vi "Receive Panel Close Event.vi"(8 "error in (no error)":errorcluster, 10 "PanelCloseMsg":refnum<class "PanelCloseMsg.lvclass">, 11 "OneButtonDialogBox in":refnum<class "OneButtonDialogBox.lvclass">) -> (0 "error out":errorcluster, 3 "OneButtonDialogBox out":refnum<class "OneButtonDialogBox.lvclass">)   [LabVIEW 2015, in "OneButtonDialogBox.lvlib" / "OneButtonDialogBox.lvclass"]
doc: "<License>\nCopyright © 2017 Composed Systems, LLC | All rights reserved\nwww.composed.io\n\nAuthor: Ethan Stern <ethan.stern@composed.io>\n\nThis software is provided \"AS IS\" WITHOUT WARRANTIES, either express or implied, AND IS FOR EDUCATIONAL PURPOSES ONLY.\n</License>"
uses:
  OneButtonDialogBox.lvclass
  Framework/ActorEvents/IEventAggregator Messages/PanelCloseMsg/PanelCloseMsg.lvclass
  <vilib>/ActorFramework/Actor/Actor.lvclass/Actor.ctl
  <vilib>/ActorFramework/Message Enqueuer/Message Enqueuer.lvclass/Message Enqueuer.ctl
  OneButtonDialogBox.lvclass/OneButtonDialogBox.ctl
  <vilib>/ActorFramework/Message Enqueuer/Init from Existing Queue.vi
  <vilib>/ActorFramework/Message Enqueuer/Enqueue.vi
  <vilib>/ActorFramework/Message Priority Queue/Priority Enqueue.vi
  <vilib>/ActorFramework/Message Enqueuer/Message Enqueuer.lvclass
  <vilib>/ActorFramework/Stop Msg/Stop Msg.lvclass
  Framework/IDialogBox/IDialogBox Messages/Dialog Return Msg/Dialog Return Msg.lvclass
  <vilib>/ActorFramework/Actor/Actor.lvclass
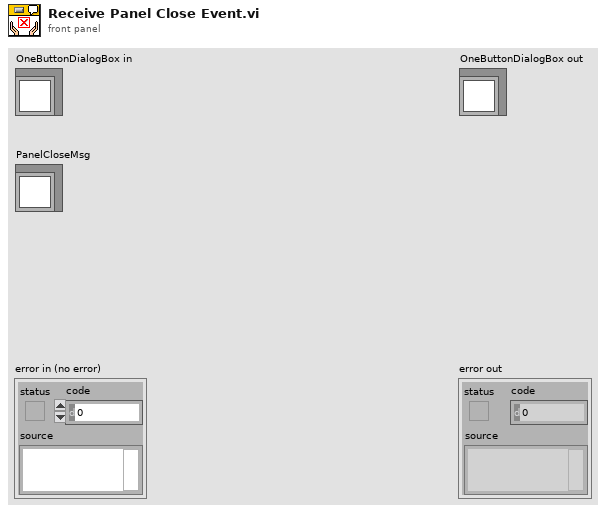
[diagram p1: front panel]
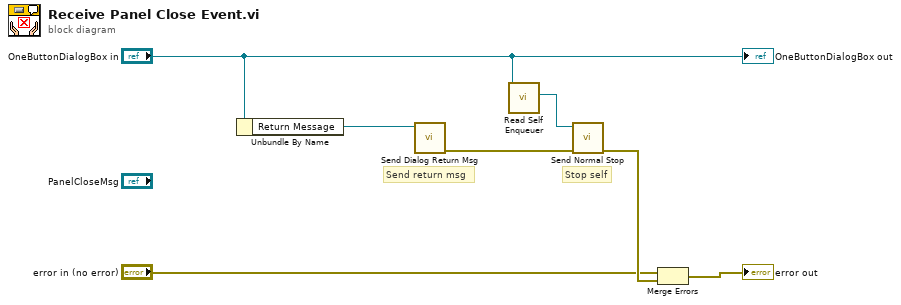
[diagram p0: block diagram]
diagram:
  # "Stop self"
  # "Send return msg"
  n1 = Unbundle By Name("OneButtonDialogBox in") -> ("Return Message"=w1:refnum<class "Dialog Return Msg.lvclass">)
  n2 = call "Send Dialog Return Msg.vi"("Dialog Return Msg"=w1) -> ("error out"=w6:errorcluster)  [unwired: 10 in]
  n3 = call <vilib>:"Read Self Enqueuer.vi"("Actor"="OneButtonDialogBox in") -> ("Self Enqueuer"=w7:refnum<class "Message Enqueuer.lvclass">)  [unwired: 10 in]
  n4 = call <vilib>:"Send Normal Stop.vi"("error in (no error)"=w6, "Message Enqueuer"=w7) -> ("error out"=w5:errorcluster)  [unwired: 9 in]
  n5 = Merge Errors("error in (no error)", w5) -> (→"error out":errorcluster)
  "OneButtonDialogBox out" <- "OneButtonDialogBox in"
